vi "getResistanceFull.vi"(4 "V_out (V)":dbl=2.5, 5 "Uncertainty (%) Vin":dbl=1.0, 6 "Uncertainty (%) Temp in":dbl=1.0, 7 "Uncertainty (%) Resistor":dbl=1.0, 8 "Temperature (K) in":dbl=300.0, 9 "V_in (V)":dbl=5.0, 10 "Uncertainty (%) Vout":dbl=1.0, 11 "Resistor (ohms)":dbl=10000.0) -> (0 "Uncertainty (%) Temp out":dbl, 1 "Temperature (K) out":dbl, 2 "Resistance":dbl, 3 "Uncertainty":dbl)   [LabVIEW 2013]
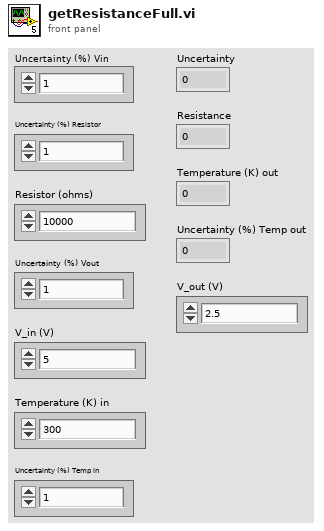
[diagram p1: front panel]
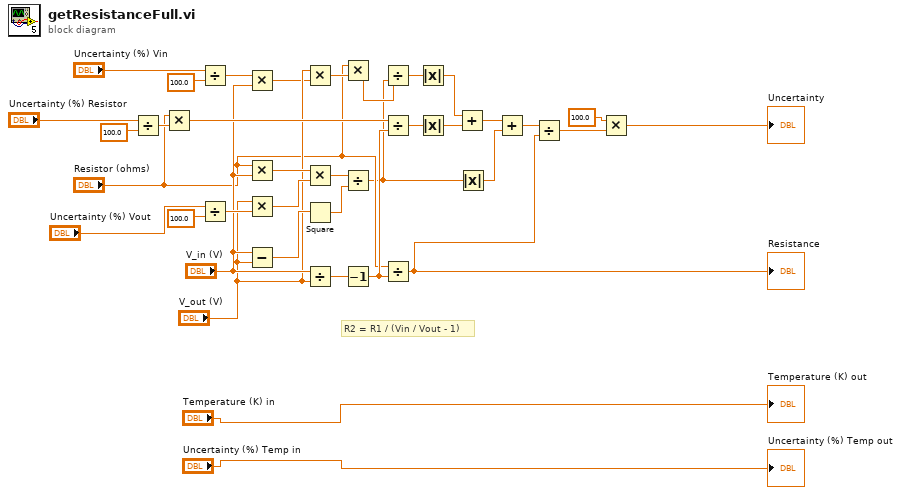
[diagram p0: block diagram]
diagram:
  # "R2 = R1 / (Vin / Vout - 1)"
  n1 = Divide(x="Uncertainty (%) Resistor", y=100.0) -> (x/y=w23:dbl)
  n2 = Multiply(x="Resistor (ohms)", y=w23) -> (x*y=w30:dbl)
  n3 = Divide(x="Uncertainty (%) Vin", y=100.0) -> (x/y=w15:dbl)
  n4 = Divide(x="Uncertainty (%) Vout", y=100.0) -> (x/y=w19:dbl)
  n5 = Multiply(x=w15, y="V_in (V)") -> (x*y=w13:dbl)
  n6 = Multiply(x="Resistor (ohms)", y="V_in (V)") -> (x*y=w28:dbl)
  n7 = Multiply(x="V_out (V)", y=w19) -> (x*y=w27:dbl)
  n8 = Subtract(x="V_in (V)", y="V_out (V)") -> (x-y=w29:dbl)
  n9 = Multiply(x="V_out (V)", y=w13) -> (x*y=w12:dbl)
  n10 = Multiply(x=w28, y=w27) -> (x*y=w26:dbl)
  n11 = Square(x=w29) -> (x^2=w25:dbl)
  n12 = Divide(x="V_in (V)", y="V_out (V)") -> (x/y=w33:dbl)
  n13 = Multiply(x="Resistor (ohms)", y=w12) -> (x*y=w10:dbl)
  n14 = Divide(x=w26, y=w25) -> (x/y=w9:dbl)
  n15 = Decrement(x=w33) -> (x-1=w32:dbl)
  n16 = Divide(x=w10, y=w9) -> (x/y=w8:dbl)
  n17 = Divide(x=w30, y=w32) -> (x/y=w31:dbl)
  n18 = Divide(x="Resistor (ohms)", y=w32) -> (x/y=w35:dbl)
  "Resistance" <- w35
  n19 = Absolute Value(x=w8) -> (abs(x)=w7:dbl)
  n20 = Absolute Value(x=w31) -> (abs(x)=w6:dbl)
  n21 = Add(x=w7, y=w6) -> (x+y=w5:dbl)
  n22 = Absolute Value(x=w9) -> (abs(x)=w4:dbl)
  n23 = Add(x=w5, y=w4) -> (x+y=w3:dbl)
  n24 = Divide(x=w3, y=w35) -> (x/y=w1:dbl)
  n25 = Multiply(x=100.0, y=w1) -> (x*y=→"Uncertainty":dbl)
  "Uncertainty (%) Temp out" <- "Uncertainty (%) Temp in"
  "Temperature (K) out" <- "Temperature (K) in"
